vi "SensorInterrupt.vi"(11 "IRQ Number":u8) -> ()   [LabVIEW 2021]
uses:
  Global 1.vi
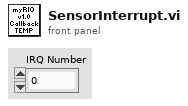
[diagram p1: front panel]
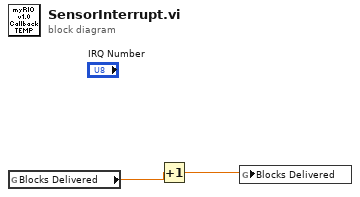
[diagram p0: block diagram]
diagram:
  n1 = global read "Global 1.vi" "Blocks Delivered"() -> (w1:dbl)
  n2 = Increment(x=w1) -> (x+1=w2:dbl)
  n3 = global write "Global 1.vi" "Blocks Delivered"(w2) -> ()
